vi "Do Update UI Event.vi"(7 "MulticolumnListbox in":refnum<vi>, 8 "error in":errorcluster, 11 "Update UI Data":variant) -> (0 "error out":errorcluster)   [LabVIEW 2016, in "Assert API Components.lvlib" / "Assert Display.lvlib" / "Main Display.lvlib" / "Main Display.lvclass"]
uses:
  Main Display.lvclass
  Components/Display Data.ctl
  Display Colours.ctl
  Main Display.lvlib
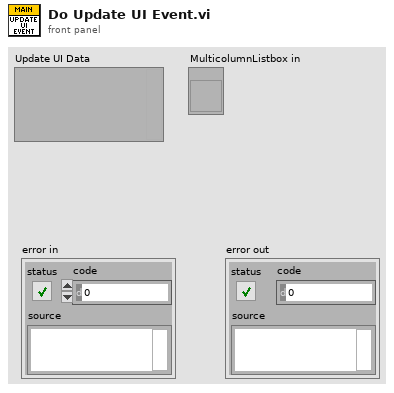
[diagram p1: front panel]
types:
  T1 = typedef "Assert API Components.lvlib/Assert Display.lvlib/Main Display.lvlib/Display Data.ctl" = cluster{"ItemNames":string[][], "Pass Fail Status":bool[], "Display Colours":T2}
  T2 = typedef "Assert API Components.lvlib/Assert Display.lvlib/Main Display.lvlib/Display Colours.ctl" = cluster{"Enable Colours":bool, "Passed Colour":u32, "Failed Colour":u32}
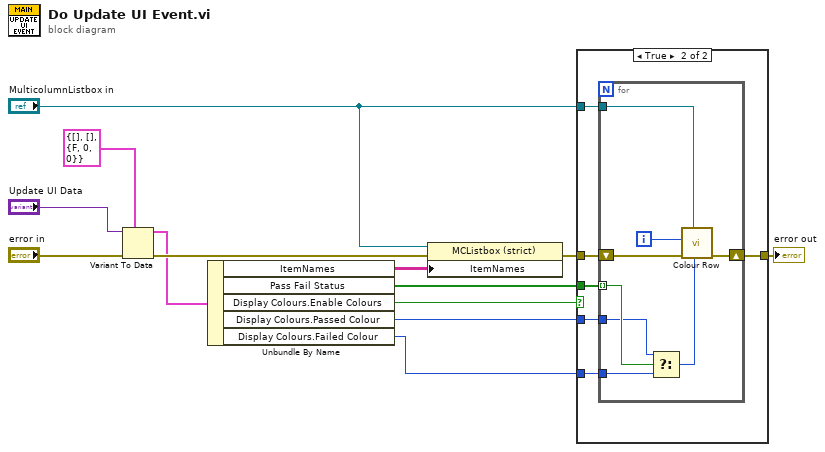
[diagram p0: block diagram]
diagram:
  n1 = Variant To Data(error in="error in", type=T1 {"ItemNames"=[], "Pass Fail Status"=[], "Display Colours"={"Enable Colours"=FALSE, "Passed Colour"=0, "Failed Colour"=0}}, Variant="Update UI Data") -> (data=w8:T1, error out=w12:errorcluster)
  n2 = Unbundle By Name(w8) -> ("ItemNames"=w7:string[][], "Pass Fail Status"=w5:bool[], "Display Colours.Enable Colours"=w4:bool, "Display Colours.Passed Colour"=w3:u32, "Display Colours.Failed Colour"=w2:u32)
  n3 = property on="Property Node" class="MCListbox (strict)"(reference="MulticolumnListbox in", error in=w12, "ItemNames"=w7) -> (error out=w13:errorcluster)  [unwired: 1 out]
  n4 = case shown="True" w4 {
    tunnel: w13 -> [w14 w17]
    tunnel: [w14 w15] -> w6
    tunnel: w5 -> [_ w20]
    tunnel: w3 -> [_ w19]
    tunnel: w2 -> [_ w18]
    tunnel: "MulticolumnListbox in" -> [_ w16]
    frame False {
    }
    frame True {
      n5 = for {
        tunnel: w20 -> [w28] mode=indexing
        tunnel: w19 -> [w27]
        tunnel: w18 -> [w26]
        shift-right: [w24] -> w15
        shift-left: w17 -> [w25]
        tunnel: w16 -> [w21]
        i -> [w23]
        n6 = Select(t=w27, s=w28, f=w26) -> (s? t:f=w22:u32)
        n7 = call "Colour Row.vi"("Row Colour"=w22, "MulticolumnListbox in"=w21, "error in (no error)"=w25, "Row Number"=w23) -> ("error out"=w24:errorcluster)  [unwired: 7 in]
      }
    }
  }
  "error out" <- w6
